vi "Create.vi"(7 "Request Options":T1, 8 "error in (no error)":errorcluster, 9 "Region":T3, 10 "AWS Credentials":T4, 11 "ARN in":refnum<class "ARN.lvclass">) -> (0 "error out":errorcluster, 3 "ARN out":refnum<class "ARN.lvclass">)   [LabVIEW 2015, in "NI_AWS_Core.lvlib" / "ARN.lvclass"]
uses:
  ARN.lvclass
  HTTP Request/AWS Credentials.ctl
  HTTP Request/Region.ctl
  HTTP Request/Request Options.ctl
  HTTP Request/Name Value Pair.ctl
  HTTP Request/HTTP Request.lvclass/HTTP Request.ctl
  ARN.lvclass/ARN.ctl
  HTTP Request/Write Credentials.vi
  HTTP Request/Write Region.vi
  HTTP Request/Write Service.vi
  HTTP Request/Write Verify Server.vi
  Write ARN.vi
  HTTP Request/HTTP Request.lvclass
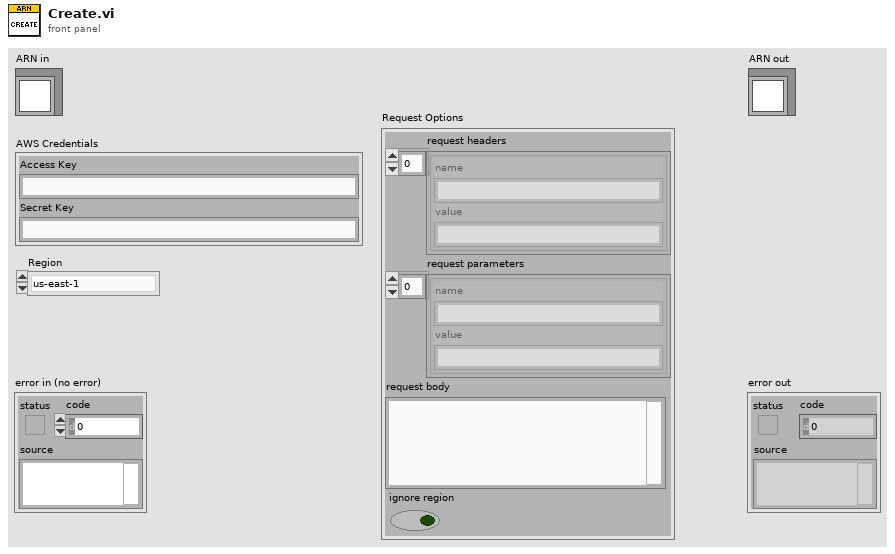
[diagram p1: front panel]
types:
  T1 = typedef "NI_AWS_Core.lvlib/HTTP Request.lvclass/Request Options.ctl" = cluster{"request headers":T2[], "request parameters":T2[], "request body":string, "ignore region":bool}
  T2 = typedef "NI_AWS_Core.lvlib/HTTP Request.lvclass/Name Value Pair.ctl" = cluster{"name":string, "value":string}
  T3 = typedef "NI_AWS_Core.lvlib/HTTP Request.lvclass/Region.ctl" = enum16{"us-east-1", "us-east-2", "us-west-1", "us-west-2", "ap-northeast-1", "ap-northeast-2", "ap-southeast-1", "ap-southeast-2", "ca-central-1", "eu-central-1", "eu-west-1", "eu-west-2", "sa-east-1"}
  T4 = typedef "NI_AWS_Core.lvlib/HTTP Request.lvclass/AWS Credentials.ctl" = cluster{"Access Key":string, "Secret Key":string}
  T5 = typedef "NI_AWS_Core.lvlib/HTTP Request.lvclass/Response.ctl" = cluster{"Headers":string, "Body":string}
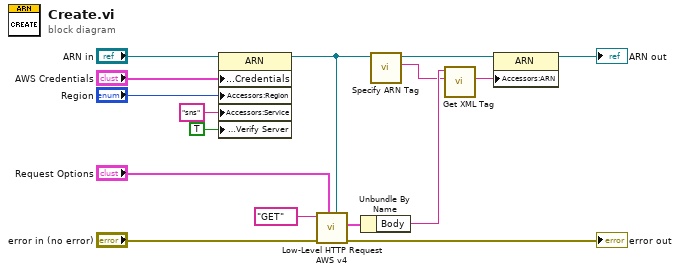
[diagram p0: block diagram]
diagram:
  n1 = property class="ARN"(reference="ARN in", "Accessors:Credentials"="AWS Credentials", "Accessors:Region"="Region", "Accessors:Service"="sns" ("Service"), "Accessors:Verify Server"=TRUE ("Verify Server")) -> (reference out=w3:refnum<class "ARN.lvclass">)  [unwired: 1 in, 1 out]
  n2 = call "Low-Level HTTP Request AWS v4.vi"("AWS Core"=w3, "Request Options"="Request Options", "error in (no error)"="error in (no error)", "HTTP-Verb"="GET") -> ("error out"=→"error out":errorcluster, "Response"=w14:T5)  [unwired: 5 in, 1 out]
  n3 = Unbundle By Name(w14) -> ("Body"=w15:string)
  n4 = call-dynamic "Specify ARN Tag.vi"("ARN in"=w3) -> ("ARN Tag"=w1:string, "ARN out"=w2:refnum<class "ARN.lvclass">)  [unwired: 9 in]
  n5 = call "Get XML Tag.vi"("Tag name"=w1, "XML String in"=w15) -> ("Tag value"=w9:string)  [unwired: 5 in, 4 out]
  n6 = property class="ARN"(reference=w2, "Accessors:ARN"=w9) -> (reference out=→"ARN out":refnum<class "ARN.lvclass">)  [unwired: 1 in, 1 out]
